vi "Measure.vi"(8 "error in (no error)":errorcluster, 9 "measurement configuration":variant, 10 "measure call context in":refnum<class "Measure Call Context.lvclass">, 11 "measurement plugin in":refnum<class "Example Plugin.lvclass">) -> (0 "error out":errorcluster, 1 "measurement results":variant, 2 "measure call context out":refnum<class "Measure Call Context.lvclass">, 3 "measurement plugin out":refnum<class "Example Plugin.lvclass">)   [LabVIEW 2025, in "Example Plugin.lvclass"]
uses:
  Example Plugin.lvclass
  <vilib>/Plug-In SDKs/Measurements/Measure Call Context/Measure Call Context.lvclass
  Measurement Configuration.ctl
  Example Plugin.lvclass/Example Plugin.ctl
  OOB Data Transfer/OOB Data Transfer.lvlib
  OOB gRPC Server/OOB gRPC Server.lvlib
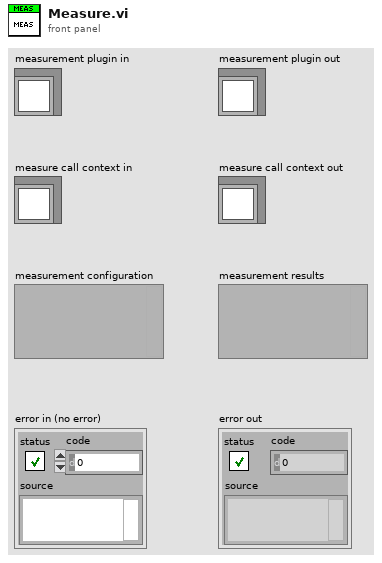
[diagram p1: front panel]
types:
  T1 = typedef "Example Plugin.lvclass/Measurement Configuration.ctl" = cluster{"Config Number":dbl, "Config String":string}
  T2 = typedef "Example Plugin.lvclass/Measurement Results.ctl" = cluster{"Config Number (Loopback)":dbl, "Config String (Loopback)":string, "Measurement Logic Counter":i32, "OOB gRPC Port":i32, "PauseResume (Loopback)":bool, "Export (Loopback)":string}
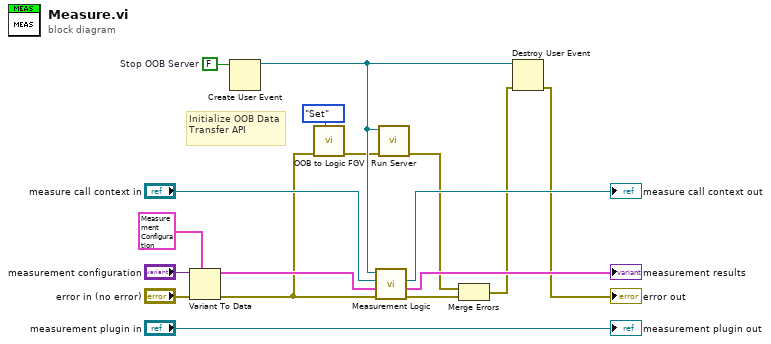
[diagram p0: block diagram]
diagram:
  w6 = FALSE  # Stop OOB Server
  # "Initialize OOB Data Transfer API"
  n1 = Variant To Data(error in="error in (no error)", type=T1 {"Config Number"=1.2, "Config String"="Lorem ipsum dolor sit"} ("measurement configuration"), Variant="measurement configuration") -> (data=w9:T1, error out=w8:errorcluster)
  n2 = Create User Event(user event datatype=w6) -> (user event=w3:refnum<user-event>)  [unwired: 1 in, 1 out]
  n3 = call "OOB to Logic FGV.vi"("Op (Get)"=enum16{"Get", "Set"}."Set", "error in (no error)"=w8) -> ("error out"=w2:errorcluster)  [unwired: 8 in, 1 out]
  n4 = call "Measurement Logic.vi"("error in"=w8, "measurement configuration"=w9, "measure call context in"="measure call context in", "Stop OOB Server UE"=w3) -> ("error out"=w17:errorcluster, "measurement results"=→"measurement results":T2, "measure call context out"=→"measure call context out":refnum<class "Measure Call Context.lvclass">)  [unwired: 5 in]
  n5 = call "Run Server.vi"("error in (no error)"=w2, "Stop OOB Server UE"=w3) -> ("error out"=w7:errorcluster)  [unwired: 9 in]
  n6 = Merge Errors(w7, w17) -> (w5:errorcluster)
  n7 = Destroy User Event(user event=w3, error in=w5) -> (error out=→"error out":errorcluster)
  "measurement plugin out" <- "measurement plugin in"
